vi "set-figure-display-names.vi"(6 "DisplayNames":string[](array[string]), 8 "error in":errorcluster, 11 "figure (in)":refnum<vi>) -> (0 "error out":errorcluster, 3 "figure (out)":refnum<vi>)   [LabVIEW 2017]
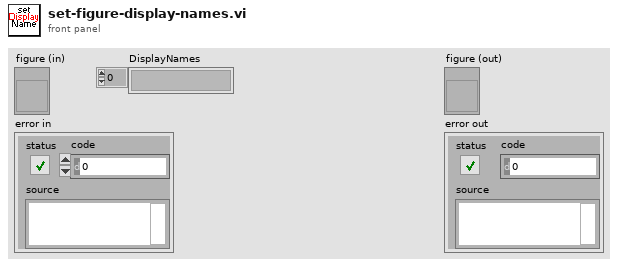
[diagram p1: front panel]
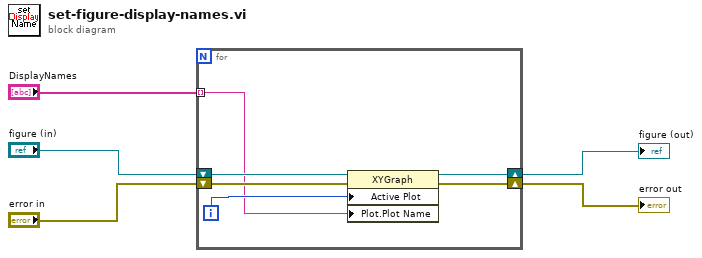
[diagram p0: block diagram]
diagram:
  n1 = for {
    shift-right: [w11] -> w5
    shift-left: "figure (in)" -> [w10]
    shift-right: [w9] -> w4
    shift-left: "error in" -> [w7]
    tunnel: "DisplayNames" -> [w6] mode=indexing
    i -> [w8]
    n2 = property class="XYGraph"(reference=w10, error in=w7, "Active Plot"=w8, "Plot.Plot Name"=w6) -> (reference out=w11:refnum<vi>, error out=w9:errorcluster)
  }
  "figure (out)" <- w5
  "error out" <- w4
